vi "Initialize.vi"(8 "error in (no error)":errorcluster, 11 "BT in":refnum<class "BT.lvclass">) -> (0 "error out":errorcluster, 3 "BT out":refnum<class "BT.lvclass">)   [LabVIEW 2014, in "BT.lvlib" / "BT.lvclass"]
uses:
  BT.lvclass
  C:/Users/yang/Desktop/BT Connect/InTheHand.Net.Personal.dll
  BT Connect/InTheHand.Net.Personal.dll
  BT.lvclass/BT.ctl
panel:
  in  "Bluetooth Service":refnum<k24>
  in  "Bluetooth Security":refnum<k24>
  in  "System.Timespan":refnum<k24>
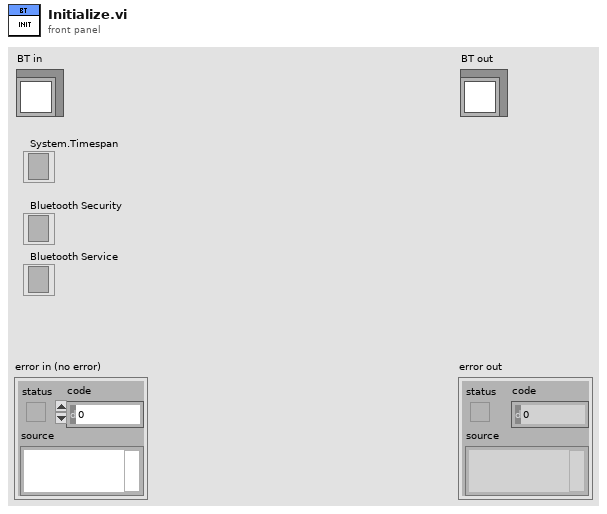
[diagram p1: front panel]
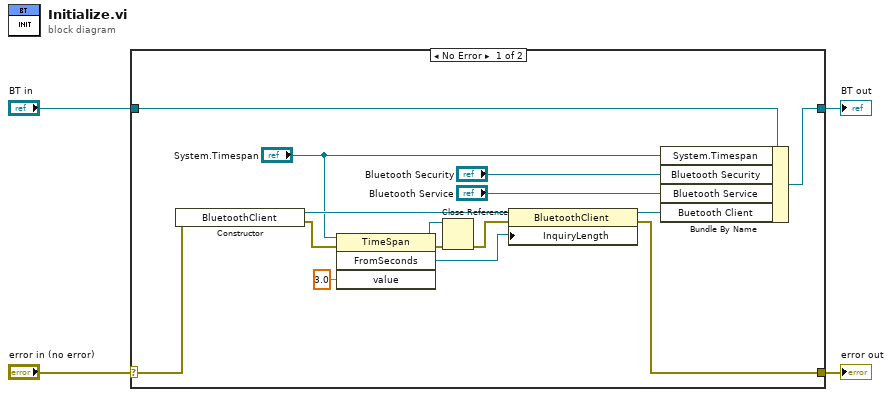
[diagram p0: block diagram]
diagram:
  n1 = case shown="No Error" "error in (no error)" {
    selector: "error in (no error)" -> [w5 w21]
    tunnel: [w6 w21] -> w3
    tunnel: [w16 w20] -> w1
    tunnel: "BT in" -> [w17 w20]
    frame No Error {
      n2 = constructor class="BluetoothClient"(error in=w5) -> (reference out=w10:refnum<k24>, error out=w8:errorcluster)  [unwired: 2 in, 1 out]
      n3 = invoke class="TimeSpan" method="FromSeconds"(reference="System.Timespan", error in=w8, "value"=3.0) -> (reference out=w13:refnum<k24>, error out=w14:errorcluster, "FromSeconds"=w11:refnum<k24>)  [unwired: 1 in, 1 out]
      n4 = Close Reference(reference=w13, error in (no error)=w14) -> (error out=w12:errorcluster)
      n5 = property class="BluetoothClient"(reference=w10, error in=w12, "InquiryLength"=w11) -> (reference out=w7:refnum<k24>, error out=w6:errorcluster)
      n6 = Bundle By Name(cluster=w17, "System.Timespan"="System.Timespan", "Bluetooth Security"="Bluetooth Security", "Bluetooth Service"="Bluetooth Service", "Buetooth Client"=w7) -> (w16:refnum<class "BT.lvclass">)
    }
    frame Error {
    }
  }
  "error out" <- w3
  "BT out" <- w1
